vi "Init.vi"(8 "error in (no error)":errorcluster, 9 "SA Pin":string, 10 "Measurement Name":string) -> (0 "error out":errorcluster, 3 "WCDMA_OBW out":refnum<class "WCDMA_OBW.lvclass">)   [LabVIEW 2016, in "SeqAuto Evaluations.lvlib" / "WCDMA_OBW.lvclass"]
uses:
  WCDMA_OBW.lvclass
  C:/Sequence Automation/Plugins/SeqAuto IEvaluation.lvlibp/SeqAuto IEvaluation.lvclass
  WCDMA_OBW.lvclass/WCDMA_OBW.ctl
  Write SA Pin.vi
  Plugins/SeqAuto IEvaluation.lvlibp/Write Measurement Name.vi
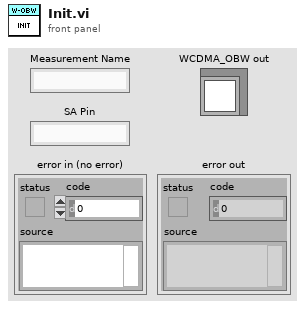
[diagram p1: front panel]
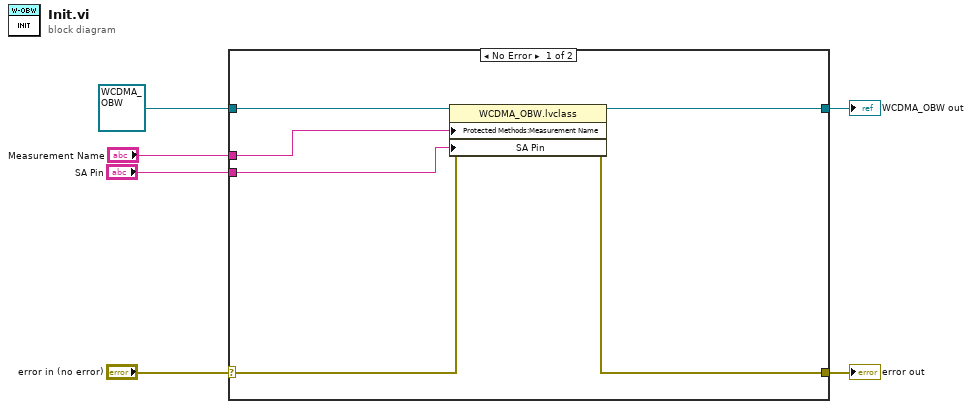
[diagram p0: block diagram]
diagram:
  n1 = case shown="No Error" "error in (no error)" {
    selector: "error in (no error)" -> [w12 w14]
    tunnel: [w11 w14] -> w5
    tunnel: [w9 w13] -> w3
    tunnel: refnum<class "WCDMA_OBW.lvclass"> refnum ("WCDMA_OBW in") -> [w10 w13]
    tunnel: "Measurement Name" -> [w8 _]
    tunnel: "SA Pin" -> [w7 _]
    frame No Error {
      n2 = property class="WCDMA_OBW.lvclass"(reference=w10, error in=w12, "Protected Methods:Measurement Name"=w8, "SA Pin"=w7) -> (reference out=w9:refnum<class "WCDMA_OBW.lvclass">, error out=w11:errorcluster)
    }
    frame Error {
    }
  }
  "error out" <- w5
  "WCDMA_OBW out" <- w3
